vi "InitRobot_SE.vi"(7 "Camera Name":refnum<k21>="cam0" caption="IMAQdx Session", 8 "VISA resource name":refnum<visa-resource-name>, 9 "Data Highway In":T1={"New Image"=refnum, "Session Out"="", "LIDAR VISA Name"="", "Phidget Device Out"=0, "Lidar Data"=[], "polar attributes"={"maximum"=0.0, "minimum"=0.0, "clip to min"=FALSE, "log?(F)"=FALSE, "grid color"=6710886, "plot color"=65280, "fmt and prec"={"format"=enum."Decimal", "precision"=0}, "visible section"=8}, "Debug Message"="", "Servo Angles"={"Angle X"=0.0, "Angle Y"=0.0}, "ColorPlane"=refnum, "Threshold"=refnum, "PartFilt"=refnum, "Processed Image"=refnum, "Magnitude"=[], "Direction"=[]} {"polar attributes"."minimum" format="%0.2f"; "polar attributes"."maximum" format="%0.2f"}) -> (3 "Data Highway Out":T1={"New Image"=refnum, "Session Out"="", "LIDAR VISA Name"="", "Phidget Device Out"=0, "Lidar Data"=[], "polar attributes"={"maximum"=0.0, "minimum"=0.0, "clip to min"=FALSE, "log?(F)"=FALSE, "grid color"=6710886, "plot color"=65280, "fmt and prec"={"format"=enum."Decimal", "precision"=0}, "visible section"=8}, "Debug Message"="", "Servo Angles"={"Angle X"=0.0, "Angle Y"=0.0}, "ColorPlane"=refnum, "Threshold"=refnum, "PartFilt"=refnum, "Processed Image"=refnum, "Magnitude"=[], "Direction"=[]} {"polar attributes"."minimum" format="%0.2f"; "polar attributes"."maximum" format="%0.2f"}, 5 "error out":errorcluster)   [LabVIEW 2014]
uses:
  controls/Data.ctl
  <vilib>/vision/Image Controls.llb/IMAQ Image.ctl
  <vilib>/userdefined/High Color/IMAQdx.ctl
  Program Files (x86)/National Instruments/LabVIEW 2014/instr.lib/Hokuyo URG Series/Public/Initialize-Standard.vi
  <vilib>/vision/driver/NI_Vision_Acquisition_Software.lvlib
  Program Files (x86)/National Instruments/LabVIEW 2014/instr.lib/Hokuyo URG Series/Hokuyo URG Series.lvlib
panel:
  out "VISA resource name out":refnum<visa-resource-name>
  out "Device Out":i32
  # "LIDAR I/O"
  # "Camera I/O"
  # "Phidget I/O"
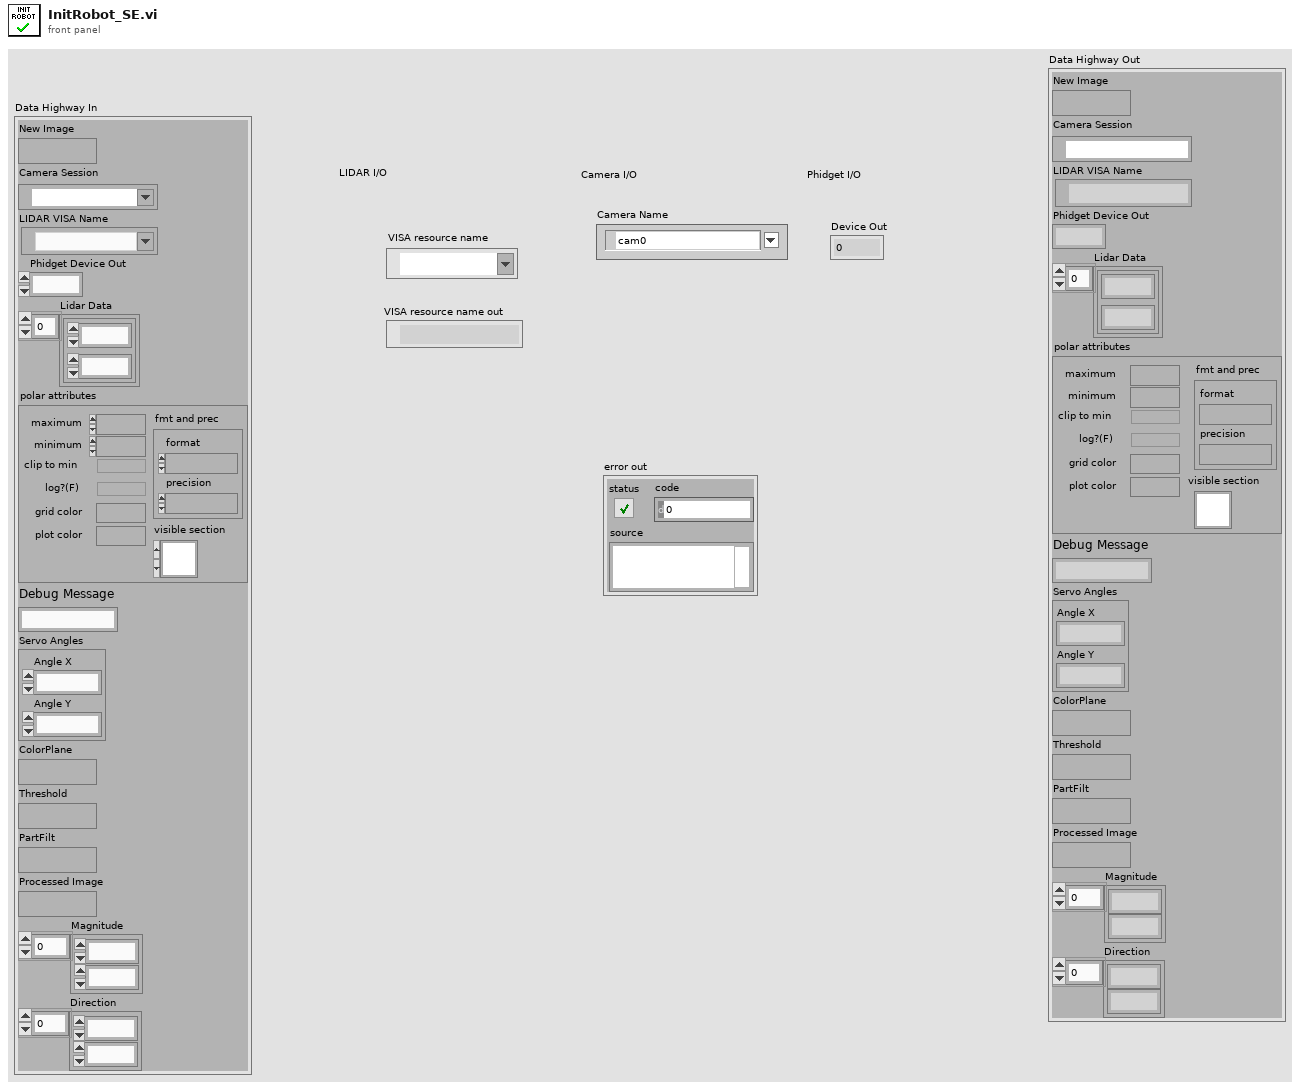
[diagram p1: front panel]
types:
  T1 = typedef "Data.ctl" = cluster{"New Image":T2, "Session Out":T3, "LIDAR VISA Name":refnum<visa-resource-name>, "Phidget Device Out":i32, "Lidar Data":cluster{dbl, dbl}[], "polar attributes":cluster{"maximum":dbl, "minimum":dbl, "clip to min":bool, "log?(F)":bool, "grid color":u32, "plot color":u32, "fmt and prec":cluster{"format":enum8{"Decimal", "Scientific", "Engineering", "Binary", "Octal", "Hex"}, "precision":u8}, "visible section":u16}, "Debug Message":string, "Servo Angles":cluster{"Angle X":dbl, "Angle Y":dbl}, "ColorPlane":T2, "Threshold":T2, "PartFilt":T2, "Processed Image":T2, "Magnitude":dbl[], "Direction":dbl[]}
  T2 = typedef "IMAQ Image.ctl" = refnum<image>
  T3 = typedef "IMAQdx.ctl" = refnum<k21>
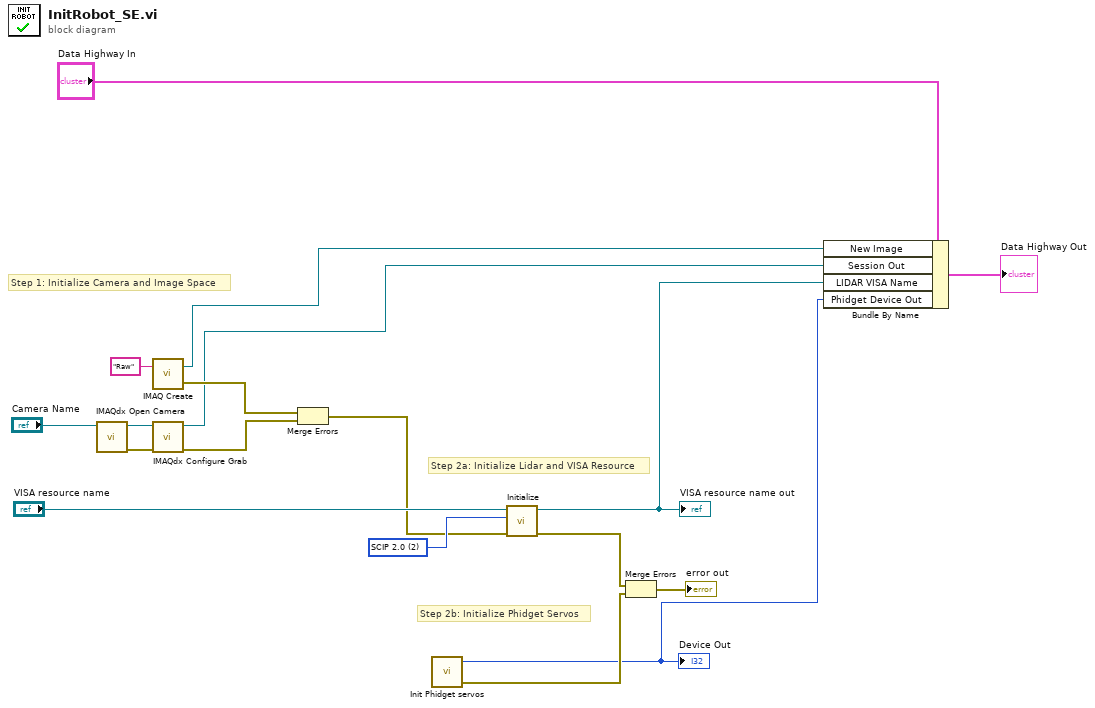
[diagram p0: block diagram]
diagram:
  w11 = u32 2 items=["Convert to Latest", "SCIP 1.1", "SCIP 2.0"] ("Protocol")
  # "Step 2b: Initialize Phidget Servos"
  # "Step 2a: Initialize Lidar and VISA Resource"
  # "Step 1: Initialize Camera and Image Space"
  n1 = call <vilib>:"IMAQdx Open Camera.vi"("Session In"="Camera Name") -> ("error out"=w15:errorcluster, "Session Out"=w16:T3)  [unwired: 2 in, 7 out]
  n2 = call "IMAQ Create"("Image Name"="Raw") -> ("New Image"=w4:T2, "error out"=w14:errorcluster)  [unwired: 3 in, 1 out]
  n3 = call <vilib>:"IMAQdx Configure Grab.vi"("error in"=w15, "Session In"=w16) -> ("error out"=w13:errorcluster, "Session Out"=w3:T3)  [unwired: 8 out]
  n4 = Merge Errors(w14, w13) -> (w10:errorcluster)
  n5 = call "Init Phidget servos.vi"() -> ("Device Out"=w1:i32, "error out"=w8:errorcluster)  [unwired: 1 in, 1 out]
  "Device Out" <- w1
  n6 = call-poly "Initialize.vi"("error in (no error)"=w10, "Protocol (2: SCIP 2.0)"=w11, "VISA resource name"="VISA resource name") -> ("error out"=w9:errorcluster, "VISA resource name out"=w2:refnum<visa-resource-name>)  [unwired: 7 in]
  "VISA resource name out" <- w2
  n7 = Merge Errors(w9, w8) -> (→"error out":errorcluster)
  n8 = Bundle By Name(cluster="Data Highway In", "New Image"=w4, "Session Out"=w3, "LIDAR VISA Name"=w2, "Phidget Device Out"=w1) -> (→"Data Highway Out":T1)
